vi "tearDown.vi"(8 "error in (no error)":errorcluster, 11 "reference in":refnum<class "[Test Case] Put and Get file.lvclass">) -> (0 "error out":errorcluster, 3 "reference out":refnum<class "[Test Case] Put and Get file.lvclass">)   [LabVIEW 2016, in "Tests.lvlib" / "[Test Case] Put and Get file.lvclass"]
doc: "tearDown runs after the test method has completed. Use this method to clean up any operations or references that were opened by setUp or the test method. Unit tests should be independent of other unit tests so this VI should ensure that the next test can run in a 'clean' test environment."
uses:
  [Test Case] Put and Get file.lvclass
  [Test Case] Put and Get file.lvclass/[Test Case] Put and Get file.ctl
  classes/File Transfer Behavior/File Transfer Behavior.lvclass
  Tests.lvlib
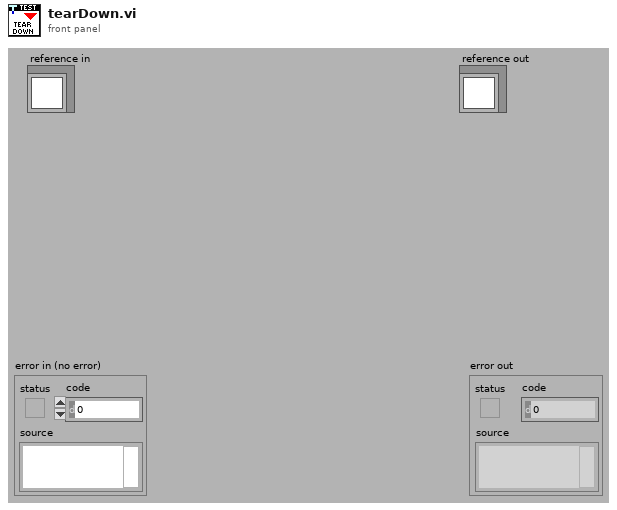
[diagram p1: front panel]
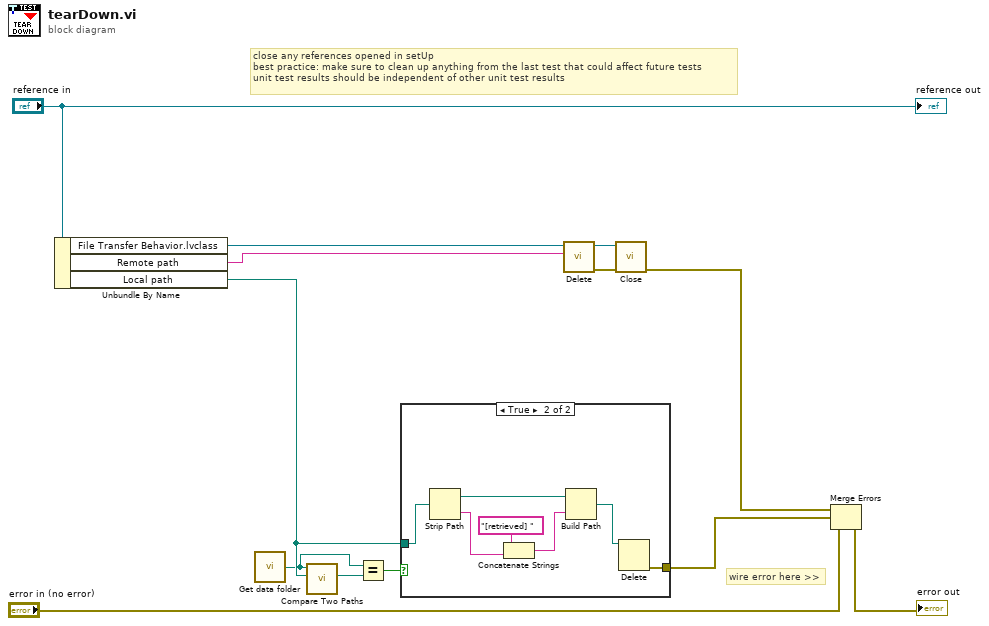
[diagram p0: block diagram]
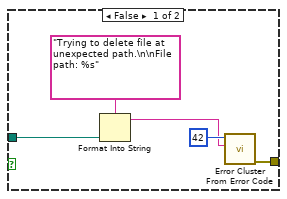
[diagram p2: hidden frame]
diagram:
  # "wire error here >>"
  # "close any references opened in setUp\nbest practice: make sure to clean up anything from the last test that could affect future tests\nunit test results should be independent of other unit test results"
  n1 = Unbundle By Name("reference in") -> ("File Transfer Behavior.lvclass"=w9:refnum<class "File Transfer Behavior.lvclass">, "Remote path"=w8:string, "Local path"=w4:path)
  n2 = call "Get data folder.vi"() -> ("Data folder"=w2:path)
  n3 = call <vilib>:"Compare Two Paths.vi"("Path 2"=w4, "Path 1"=w2) -> ("Common Path"=w3:path)  [unwired: 6 in, 3 out]
  n4 = Equal?(x=w2, y=w3) -> (x = y?=w1:bool)
  n5 = case shown="True" w1 {
    tunnel: [w18 w25] -> w5
    tunnel: w4 -> [w15 w20]
    frame False {
      n6 = Format Into String(format string="Trying to delete file at unexpected path.\n\nFile path: %s" ("error message (\"\")"), w15) -> (resulting string=w14:string)  [unwired: 2 in, 1 out]
      n7 = call <vilib>:"Error Cluster From Error Code.vi"("error message (\"\")"=w14, "error code (0)"=42) -> ("error out"=w18:errorcluster)  [unwired: 7 in]
    }
    frame True {
      n8 = Strip Path(path=w20) -> (stripped path=w21:path, name=w24:string)
      n9 = Concatenate Strings("[retrieved] " ("string"), w24) -> (w23:string)
      n10 = Build Path(base path=w21, name or relative path=w23) -> (appended path=w19:path)
      n11 = Delete(path (use dialog)=w19) -> (error out=w25:errorcluster)  [unwired: 4 in, 2 out]
    }
  }
  n12 = call-dynamic "Delete.vi"("Path"=w8, "File Transfer Behavior in"=w9) -> ("error out"=w11:errorcluster, "File Transfer Behavior out"=w10:refnum<class "File Transfer Behavior.lvclass">)  [unwired: 8 in]
  n13 = call-dynamic "Close.vi"("error in (no error)"=w11, "File Transfer Behavior in"=w10) -> ("error out"=w7:errorcluster)  [unwired: 9 in]
  n14 = Merge Errors(w7, w5, "error in (no error)") -> (→"error out":errorcluster)
  "reference out" <- "reference in"
